vi "Set logging mode.vi"(1 "Logging mode":bool=TRUE, 2 "Path in":path=path "C:/PI_lvlog.txt", 3 "File dialog?":bool=TRUE, 5 "error in":errorcluster) -> (19 "error out":errorcluster)   [LabVIEW 2026]
doc: "Sets logging mode for all communication interfaces. When Logging mode is ON, each string sent to or received from the controller is written to a .txt file for debugging. When File dialog is TRUE, a dialog box will pop up where the file to write can be selected, otherwise Path in must contain a valid path to a .txt file. Depending on the call chain of Set logging mode.vi, the VI will either stop (correct behavior when called from another VI) or it will remain idle (correct behavior when command VIs from this driver set are to be run manually, i.e. non-programmatically). In the latter case do not forget to press the STOP button when you have finished working with the command VIs."
uses:
  Global1.vi
panel:
  in  "Warning":string="Please do not forget\nto stop this VI when\nyou have finished working.\nmanually with this driver set."
  out "Running":u32(colorbox)=1985280 caption="Status"
  in  "stop":bool
  out "call chain":string[](array[string])=["Analog_Configuration_Setup.vi", "Analog_Sample_Application_3.vi"]
  # "Sets logging mode for all communication interfaces. When Logging mode is ON, each \nstring sent to or received from the controller is written to a .txt file for debugging."
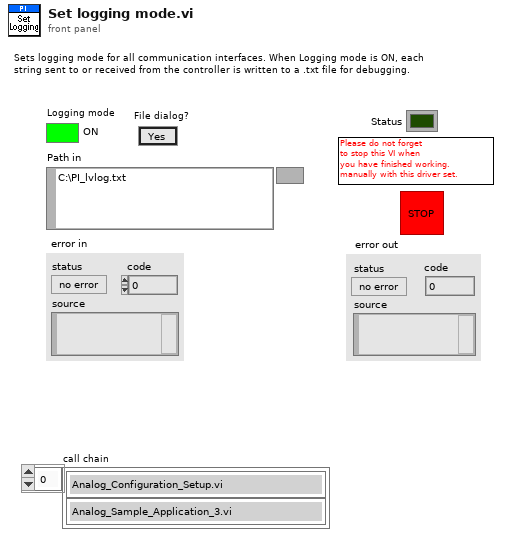
[diagram p1: front panel]
types:
  T1 = enum16{"open", "replace", "create", "open or create", "replace or create", "replace or create with confirmation"}
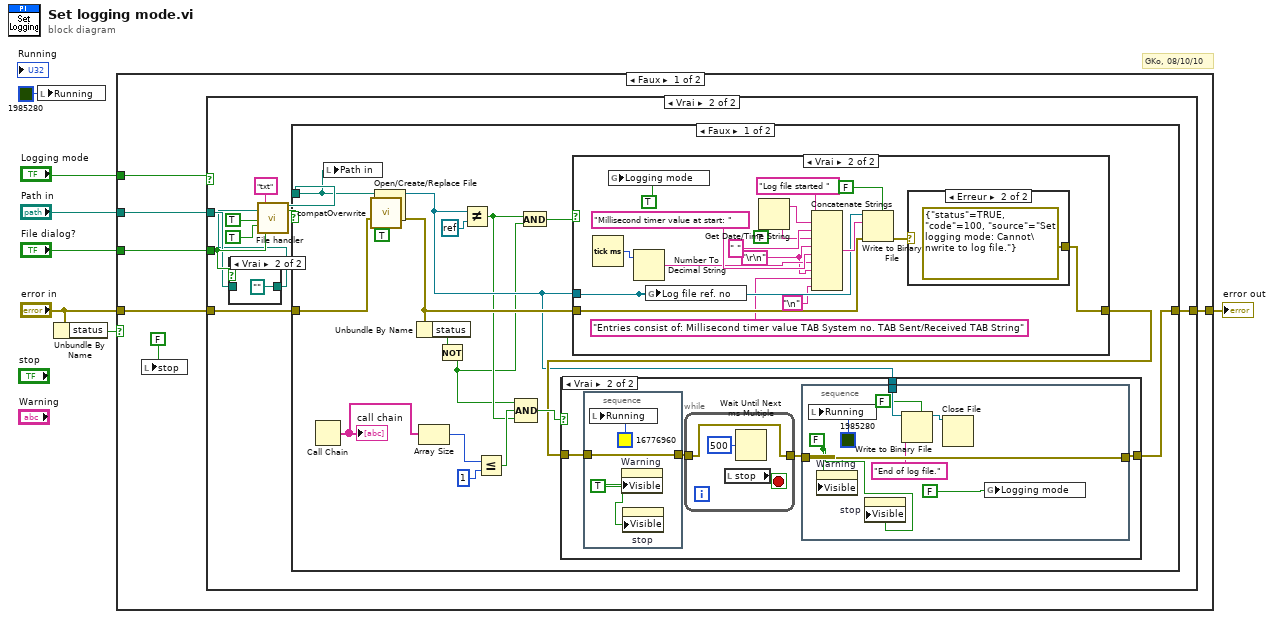
[diagram p0: block diagram]
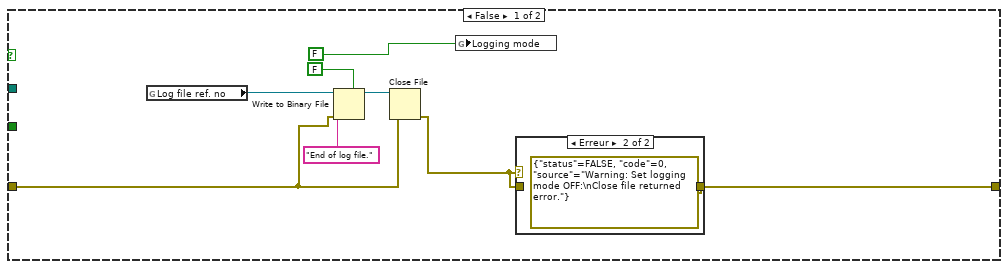
[diagram p2: hidden frame]
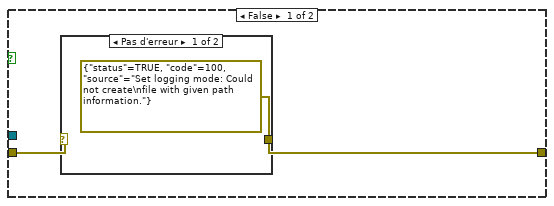
[diagram p6: hidden frame]
diagram:
  # "GKo, 08/10/10"
  n1 = local write "Running"(u32 1985280 ("Running")) -> ()
  n2 = Unbundle By Name("error in") -> ("status"=w6:bool)
  n3 = case shown="Faux" w6 {
    tunnel: [w10 w99] -> w7
    tunnel: "error in" -> [w8 w99]
    tunnel: "File dialog?" -> [w13 _]
    tunnel: "Path in" -> [w12 _]
    tunnel: "Logging mode" -> [w11 _]
    frame False {
      n4 = local write "stop"(FALSE ("stop")) -> ()
      n5 = case shown="Vrai" w11 {
        tunnel: w13 -> [_ w26]
        tunnel: w12 -> [_ w25]
        tunnel: w8 -> [w18 w28]
        tunnel: [w21 w27] -> w10
        frame False {
          n6 = global read "Global1.vi" "Log file ref. no"() -> (w16:refnum<file>)
          n7 = Write to Binary File(file (use dialog)=w16, data="End of log file." ("string"), error in=w18, 5:FALSE ("prepend array or string size? (T)")) -> (refnum out=w17:refnum<file>)  [unwired: 4 out]
          n8 = Close File(refnum=w17, error in=w18) -> (error out=w20:errorcluster)  [unwired: 1 out]
          n9 = global write "Global1.vi" "Logging mode"(FALSE ("new element/subarray")) -> ()
          n10 = case shown="Erreur" w20 {
            tunnel: w20 -> [w22 _]
            tunnel: [w22 errorcluster {"status"=FALSE, "code"=0, "source"="Warning: Set logging mode OFF:\nClose file returned error."} ("error out")] -> w21
            frame No Error {
            }
            frame Error {
            }
          }
        }
        frame True {
          n11 = case shown="Vrai" w26 {
            tunnel: w25 -> [w34 _]
            tunnel: [w34 path ""] -> w24
            frame False {
            }
            frame True {
            }
          }
          n12 = call "File handler.vi"("Path in"=w24, "Read (F) or write (T)?"=TRUE ("New File?"), "Write new File?"=TRUE, "Extension"="txt", "With dialog?"=w26) -> ("Path out"=w29:path, "Cancelled?"=w30:bool)  [unwired: 1 in, 12 out]
          n13 = case shown="Faux" w30 {
            tunnel: w29 -> [w37 _]
            tunnel: w28 -> [w52 w98]
            tunnel: [w42 w98] -> w27
            frame False {
              n14 = Call Chain() -> (call chain=w48:string[])
              "call chain" <- w48
              n15 = local write "Path in"(w37) -> ()
              n16 = call <vilib>:"compatOverwrite.vi"("overwrite (F)"=TRUE) -> ("overwrite?"=w36:T1)
              n17 = Open/Create/Replace File(file path (use dialog)=w37, error in=w52, operation (0:open)=w36) -> (refnum out=w41:refnum<file>, error out=w46:errorcluster)  [unwired: 4 out]
              n18 = Unbundle By Name(w46) -> ("status"=w45:bool)
              n19 = Array Size(array=w48) -> (size(s)=w49:i32)
              n20 = Not(x=w45) -> (.not. x?=w38:bool)
              n21 = Not Equal?(x=w41, y=refnum<k0> refnum) -> (x != y?=w40:bool)
              n22 = Less Or Equal?(x=w49, y=1) -> (x <= y?=w47:bool)
              n23 = Compound Arithmetic op=AND(w38, w47, w40) -> (w44:bool)
              n24 = And(x=w40, y=w38) -> (x .and. y?=w39:bool)
              n25 = case shown="Vrai" w39 {
                tunnel: w41 -> [_ w86]
                tunnel: w46 -> [w75 w90]
                tunnel: [w74 w88] -> w43
                frame False {
                  n26 = case shown="Pas d'erreur" w75 {
                    selector: w75 -> [_ w77]
                    tunnel: [errorcluster {"status"=TRUE, "code"=100, "source"="Set logging mode: Could not create\nfile with given path information."} ("error IO") w77] -> w74
                    frame No Error {
                    }
                    frame Error {
                    }
                  }
                }
                frame True {
                  w80 = "\r\n"
                  n27 = Tick Count (ms)() -> (millisecond timer value=w83:u32)
                  n28 = global write "Global1.vi" "Logging mode"(TRUE ("new element/subarray")) -> ()
                  n29 = Number To Decimal String(number=w83) -> (decimal integer string=w82:string)  [unwired: 1 out]
                  n30 = global write "Global1.vi" "Log file ref. no"(w86) -> ()
                  n31 = Get Date/Time String(want seconds? (F)=TRUE) -> (date string=w94:string, time string=w92:string)  [unwired: 2 out]
                  n32 = Concatenate Strings("Log file started " ("string"), w94, " ", w92, w80, "Millisecond timer value at start: " ("string"), w82, w80, "Entries consist of: Millisecond timer value TAB System no. TAB Sent/Received TAB String" ("string"), "\n" ("string")) -> (w91:string)
                  n33 = Write to Binary File(file (use dialog)=w86, data=w91, error in=w90, 5:FALSE ("prepend array or string size? (T)")) -> (error out=w89:errorcluster)  [unwired: 4 out]
                  n34 = case shown="Erreur" w89 {
                    selector: w89 -> [w96 _]
                    tunnel: [w96 errorcluster {"status"=TRUE, "code"=100, "source"="Set logging mode: Cannot\nwrite to log file."} ("error IO")] -> w88
                    frame No Error {
                    }
                    frame Error {
                    }
                  }
                }
              }
              n35 = case shown="Vrai" w44 {
                tunnel: w43 -> [w54 w58]
                tunnel: [w54 w59] -> w42
                tunnel: w41 -> [_ w55]
                frame False {
                }
                frame True {
                  n36 = stacked-sequence {
                    tunnel: w58 -> [w62]
                    tunnel: [w62] -> w57
                    frame #0 {
                      w60 = TRUE ("Visible")
                      n37 = local write "Running"(u32 16776960 ("Running")) -> ()
                      n38 = property on="Warning" class="Ch"("Visible"=w60) -> ()  [unwired: 2 in, 2 out]
                      n39 = property on="stop" class="Bool (strict)"("Visible"=w60) -> ()  [unwired: 2 in, 2 out]
                    }
                  }
                  n40 = while {
                    tunnel: w57 -> [w71]
                    tunnel: [w71] -> w56
                    stop <- w72 stop-if-true
                    n41 = local read "stop"() -> (w72:bool)
                    n42 = Wait Until Next ms Multiple(millisecond multiple=u32 500) -> ()  [unwired: 1 out]
                  }
                  n43 = stacked-sequence {
                    tunnel: w56 -> [w70]
                    tunnel: [w70] -> w59
                    tunnel: w55 -> [w68]
                    frame #0 {
                      w65 = FALSE ("Visible")
                      n44 = local write "Running"(u32 1985280 ("Running")) -> ()
                      n45 = property on="Warning" class="Ch"("Visible"=w65) -> ()  [unwired: 2 in, 2 out]
                      n46 = property on="stop" class="Bool (strict)"("Visible"=w65) -> ()  [unwired: 2 in, 2 out]
                      n47 = Write to Binary File(file (use dialog)=w68, data="End of log file." ("string"), 5:FALSE ("prepend array or string size? (T)")) -> (refnum out=w67:refnum<file>)  [unwired: 1 in, 4 out]
                      n48 = Close File(refnum=w67) -> ()  [unwired: 1 in, 2 out]
                      n49 = global write "Global1.vi" "Logging mode"(FALSE ("new element/subarray")) -> ()
                    }
                  }
                }
              }
            }
            frame True {
            }
          }
        }
      }
    }
    frame True {
    }
  }
  "error out" <- w7
